vi "GetPosition(degree).vi"(8 "error in (no error)":errorcluster, 11 "Motor Base in":refnum<class "Motor Base.lvclass">) -> (0 "error out":errorcluster, 2 "degree":dbl, 3 "Motor Base out":refnum<class "Motor Base.lvclass">)   [LabVIEW 2016, in "Motor Base.lvlib" / "Motor Base.lvclass"]
uses:
  Motor Base.lvclass
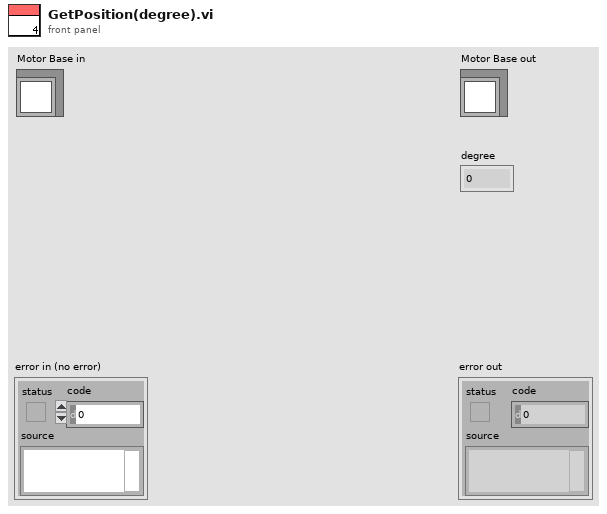
[diagram p1: front panel]
types:
  T1 = cluster{"Modes of operation":i8, "Feed(pulse)":u32, "Max motor speed(r/min)":u32, "Max torque(0.1%)":u16, "Min position limit(pulse)":i32, "Max position limit(pulse)":i32}
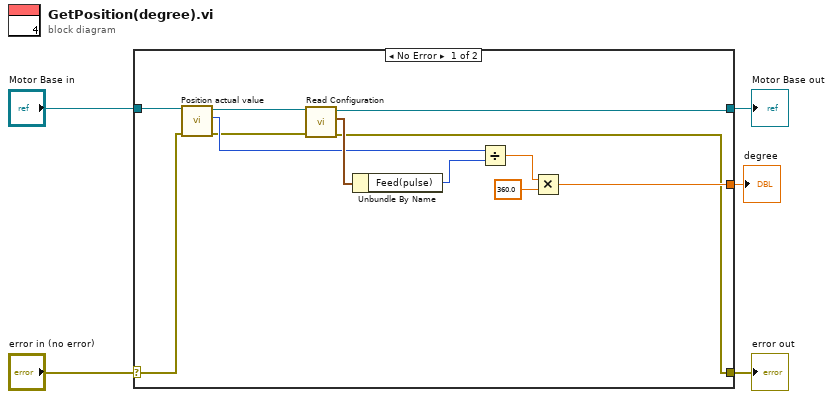
[diagram p0: block diagram]
diagram:
  n1 = case shown="No Error" "error in (no error)" {
    selector: "error in (no error)" -> [w12 w19]
    tunnel: [w6 w19] -> w4
    tunnel: [w7 w18] -> w2
    tunnel: "Motor Base in" -> [w17 w18]
    tunnel: [w8 _] -> w1
    frame No Error {
      n2 = call-dynamic "Position actual value.vi"("error in"=w12, "Motor Base in"=w17) -> ("error out"=w11:errorcluster, "Data"=w14:i32, "Motor Base out"=w16:refnum<class "Motor Base.lvclass">)  [unwired: 7 in]
      n3 = call-dynamic "Read Configuration.vi"("error in (no error)"=w11, "Motor Base in"=w16) -> ("error out"=w6:errorcluster, "Configuration"=w15:T1, "Motor Base out"=w7:refnum<class "Motor Base.lvclass">)  [unwired: 7 in]
      n4 = Unbundle By Name(w15) -> ("Feed(pulse)"=w13:u32)
      n5 = Divide(x=w14, y=w13) -> (x/y=w10:dbl)
      n6 = Multiply(x=w10, y=360.0) -> (x*y=w8:dbl)
    }
    frame Error {
    }
  }
  "error out" <- w4
  "Motor Base out" <- w2
  "degree" <- w1
